vi "Calculate Ellipse.vi"(7 "Display":bool, 9 "steps":i32=36, 10 "Ellipse":T1 {"Minor Axis"."Point 2"."Y" format="%.2f"; "Minor Axis"."Point 2"."X" format="%.2f"; "Minor Axis"."Point 1"."Y" format="%.2f"; "Minor Axis"."Point 1"."X" format="%.2f"; "Major Axis"."Point 2"."Y" format="%.2f"; "Major Axis"."Point 2"."X" format="%.2f"; "Major Axis"."Point 1"."Y" format="%.2f"; "Major Axis"."Point 1"."X" format="%.2f"; "Center"."Y" format="%.2f"; "Center"."X" format="%.2f"}) -> (1 "Effective Diameter":sgl, 2 "Ellipse Coordinates":cluster{"X":i32, "Y":i32}[](array[cluster]), 4 "y position":dbl, 6 "x position":dbl)   [LabVIEW 2013]
panel:
  out "angle":dbl
  out "b":dbl
  out "a":dbl
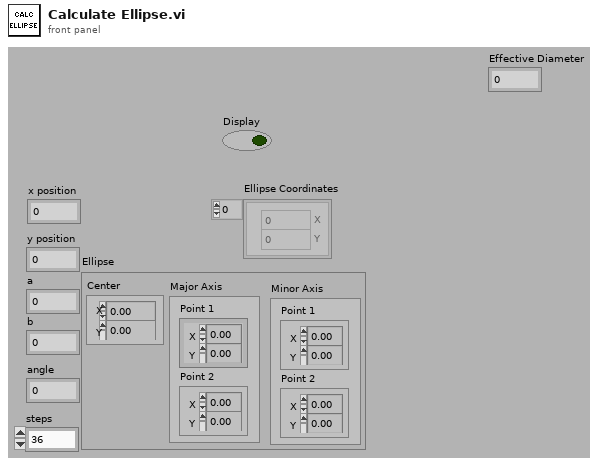
[diagram p1: front panel]
types:
  T1 = cluster{"Center":cluster{"X":sgl, "Y":sgl}, "Major Axis":cluster{"Point 1":cluster{"X":sgl, "Y":sgl}, "Point 2":cluster{"X":sgl, "Y":sgl}}, "Minor Axis":cluster{"Point 1":cluster{"X":sgl, "Y":sgl}, "Point 2":cluster{"X":sgl, "Y":sgl}}}
  T2 = cluster{"Point 1":cluster{"X":sgl, "Y":sgl}, "Point 2":cluster{"X":sgl, "Y":sgl}}
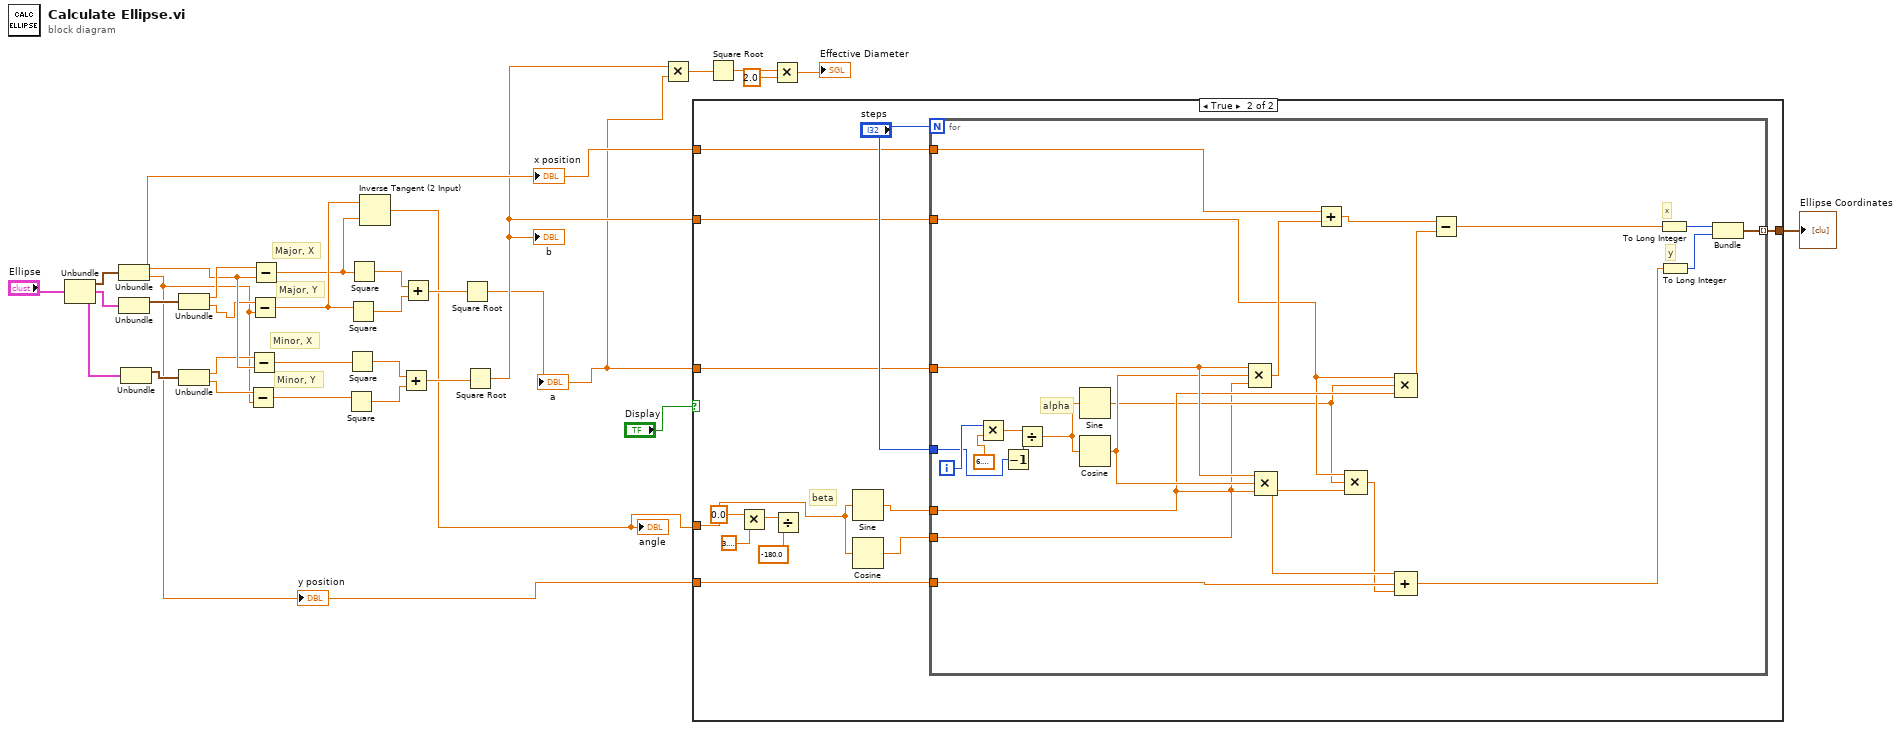
[diagram p0: block diagram]
diagram:
  # "Minor, Y"
  # "Minor, X"
  # "Major, Y"
  # "Major, X"
  n1 = Unbundle("Ellipse") -> ("Center"=w29:cluster{"X":sgl, "Y":sgl}, "Major Axis"=w28:T2, "Minor Axis"=w27:T2)
  n2 = Unbundle(w29) -> ("X"=w19:sgl, "Y"=w13:sgl)
  "x position" <- w19
  "y position" <- w13
  n3 = Unbundle(w28) -> ("Point 1"=w26:cluster{"X":sgl, "Y":sgl})  [unwired: 1 out]
  n4 = Unbundle(w27) -> ("Point 1"=w25:cluster{"X":sgl, "Y":sgl})  [unwired: 1 out]
  n5 = Unbundle(w26) -> ("X"=w24:sgl, "Y"=w14:sgl)
  n6 = Unbundle(w25) -> ("X"=w18:sgl, "Y"=w17:sgl)
  n7 = Subtract(x=w17, y=w13) -> (x-y=w22:sgl)
  n8 = Subtract(x=w18, y=w19) -> (x-y=w23:sgl)
  n9 = Subtract(x=w14, y=w13) -> (x-y=w3:sgl)
  n10 = Subtract(x=w24, y=w19) -> (x-y=w2:sgl)
  n11 = Square(x=w22) -> (x^2=w20:sgl)
  n12 = Square(x=w23) -> (x^2=w21:sgl)
  n13 = Square(x=w3) -> (x^2=w4:sgl)
  n14 = Square(x=w2) -> (x^2=w5:sgl)
  n15 = Inverse Tangent (2 Input)(1:w2, 2:w3) -> (0:w1:sgl)
  "angle" <- w1
  n16 = Add(x=w21, y=w20) -> (x+y=w16:sgl)
  n17 = Add(x=w5, y=w4) -> (x+y=w15:sgl)
  n18 = Square Root(x=w15) -> (sqrt(x)=w11:sgl)
  "a" <- w11
  n19 = Square Root(x=w16) -> (sqrt(x)=w12:sgl)
  "b" <- w12
  n20 = Multiply(x=w12, y=w11) -> (x*y=w10:sgl)
  n21 = case shown="True" "Display" {
    tunnel: [_ w44] -> w31
    tunnel: w19 -> [_ w37]
    tunnel: w1 -> [_ w33]
    tunnel: w13 -> [_ w36]
    tunnel: w12 -> [_ w35]
    tunnel: w11 -> [_ w34]
    frame False {
    }
    frame True {
      # "beta"
      n22 = Multiply(x=0.0, y=3.141592653589793) -> (x*y=w42:dbl)
      n23 = Divide(x=w42, y=-180.0) -> ()  [unwired: 1 out]
      n24 = Sine(x=w33) -> (sin(x)=w38:sgl)
      n25 = Cosine(x=w33) -> (cos(x)=w39:sgl)
      n26 = for {
        N: "steps" -> [_]
        tunnel: [w68] -> w44 mode=indexing
        tunnel: "steps" -> [w46]
        tunnel: w37 -> [w63]
        tunnel: w36 -> [w53]
        tunnel: w34 -> [w57]
        tunnel: w39 -> [w48]
        tunnel: w35 -> [w50]
        tunnel: w38 -> [w55]
        i -> [w67]
        # "y"
        # "x"
        # "alpha"
        n27 = Multiply(x=w67, y=6.283185307179586) -> (x*y=w66:dbl)
        n28 = Decrement(x=w46) -> (x-1=w45:i32)
        n29 = Divide(x=w66, y=w45) -> (x/y=w64:dbl)
        n30 = Sine(x=w64) -> (sin(x)=w49:dbl)
        n31 = Cosine(x=w64) -> (cos(x)=w56:dbl)
        n32 = Compound Arithmetic op=MULTIPLY(w57, w56, w48) -> (w62:dbl)
        n33 = Compound Arithmetic op=MULTIPLY(w57, w56, w55) -> (w54:dbl)
        n34 = Add(x=w63, y=w62) -> (x+y=w60:dbl)
        n35 = Compound Arithmetic op=MULTIPLY(w50, w49, w48) -> (w47:dbl)
        n36 = Compound Arithmetic op=MULTIPLY(w50, w49, w55) -> (w61:dbl)
        n37 = Compound Arithmetic op=ADD(w54, w53, w47) -> (w52:dbl)
        n38 = Subtract(x=w60, y=w61) -> (x-y=w59:dbl)
        n39 = To Long Integer(number=w59) -> (32bit integer=w58:i32)
        n40 = To Long Integer(number=w52) -> (32bit integer=w51:i32)
        n41 = Bundle(w58, w51) -> (w68:cluster{i32, i32})  [unwired: 1 in]
      }
    }
  }
  "Ellipse Coordinates" <- w31
  n42 = Square Root(x=w10) -> (sqrt(x)=w9:sgl)
  n43 = Multiply(x=w9, y=sgl 2.0) -> (x*y=→"Effective Diameter":sgl)
